vi "Tactic.vi"(11 "IA State Input":T1) -> (3 "IA State Output":T1)   [LabVIEW 2016]
uses:
  Core/AI Input.ctl
  Core/AI Robot.ctl
  Core/AI Ball.ctl
  Core/Field Size.ctl
  Core/AI Judge.ctl
  Command Enum.ctl
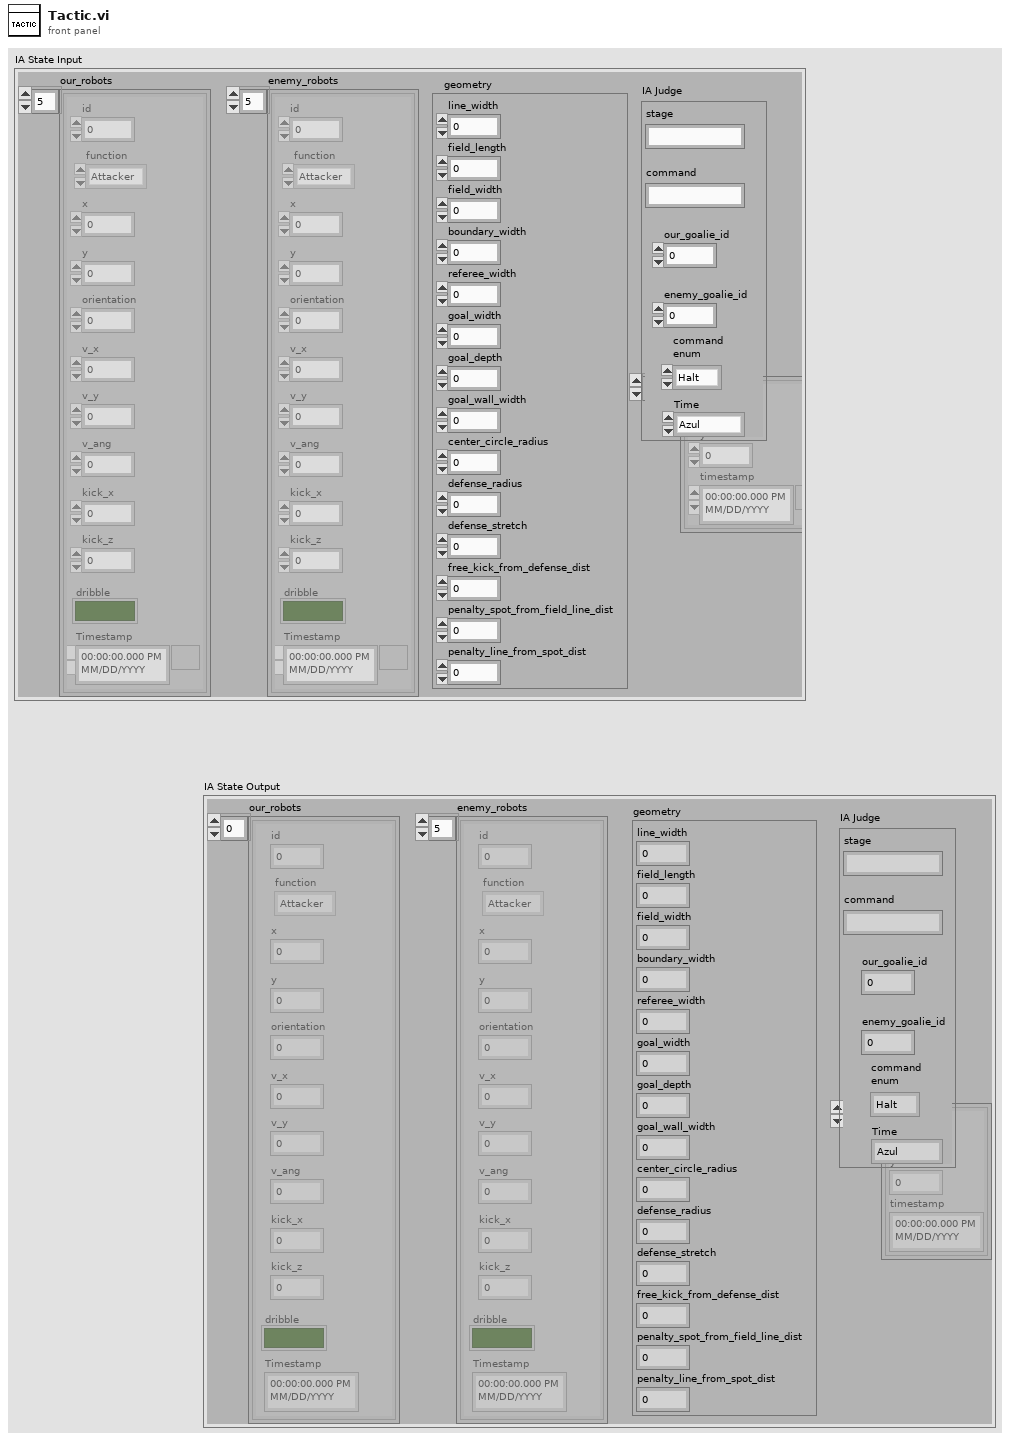
[diagram p1: front panel]
types:
  T1 = typedef "AI Input.ctl" = cluster{"our_robots":T2[], "enemy_robots":T2[], "balls":T3[], "geometry":T4, "IA Judge":T5}
  T2 = typedef "AI Robot.ctl" = cluster{"id":u32, "function":enum16{"Attacker", "Goalie", "Defender"}, "x":dbl, "y":dbl, "orientation":dbl, "v_x":dbl, "v_y":dbl, "v_ang":dbl, "kick_x":dbl, "kick_z":dbl, "dribble":bool, "Timestamp":timestamp}
  T3 = typedef "AI Ball.ctl" = cluster{"x":dbl, "y":dbl, "timestamp":timestamp}
  T4 = typedef "Field Size.ctl" = cluster{"line_width":u32, "field_length":u32, "field_width":u32, "boundary_width":u32, "referee_width":u32, "goal_width":u32, "goal_depth":u32, "goal_wall_width":u32, "center_circle_radius":u32, "defense_radius":u32, "defense_stretch":u32, "free_kick_from_defense_dist":u32, "penalty_spot_from_field_line_dist":u32, "penalty_line_from_spot_dist":u32}
  T5 = typedef "AI Judge.ctl" = cluster{"stage":string, "command":string, "our_goalie_id":dbl, "enemy_goalie_id":dbl, "command\nenum":T6, "Time":enum16{"Azul", "Amarelo"}}
  T6 = typedef "Command Enum.ctl" = enum16{"Halt", "Stop", "Force Start", "PKA Normal Start", "Prepare Kickoff Ally", "PKE Normal Start", "Prepare Kickoff Enemy", "Prepare Penalty Ally", "Prepare Penalty Enemy", "Direct Free Enemy", "Direct Free Ally", "Indirect Free Enemy", "Indirect Free Ally", "Timeout Enemy", "Timeout Ally", "Goal Enemy", "Goal Ally", "Ball Placement Enemy", "Ball Placement Ally", "None"}
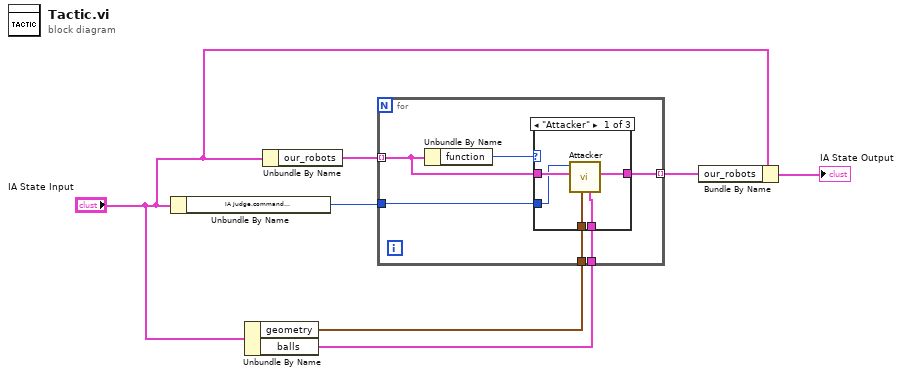
[diagram p0: block diagram]
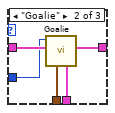
[diagram p2: hidden frame]
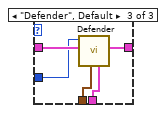
[diagram p3: hidden frame]
diagram:
  n1 = Unbundle By Name("IA State Input") -> ("IA Judge.command\nenum"=w6:T6)
  n2 = Unbundle By Name("IA State Input") -> ("geometry"=w2:T4, "balls"=w1:T3[])
  n3 = Unbundle By Name("IA State Input") -> ("our_robots"=w7:T2[])
  n4 = for {
    tunnel: w7 -> [w12] mode=indexing
    tunnel: [w11] -> w5 mode=indexing
    tunnel: w6 -> [w10]
    tunnel: w2 -> [w9]
    tunnel: w1 -> [w8]
    n5 = Unbundle By Name(w12) -> ("function"=w13:enum16{"Attacker", "Goalie", "Defender"})
    n6 = case shown="\"Attacker\"" w13 {
      tunnel: w12 -> [w18 w23 w28]
      tunnel: [w17 w22 w26] -> w11
      tunnel: w10 -> [w16 w21 w27]
      tunnel: w9 -> [w15 w19 w24]
      tunnel: w8 -> [w14 w20 w25]
      frame "Attacker" {
        n7 = call "Attacker.vi"("balls"=w14, "Field Size 2"=w15, "Robot"=w18, "command\nenum"=w16) -> ("output cluster"=w17:T2)  [unwired: 7 in]
      }
      frame "Goalie" {
        n8 = call "Goalie.vi"("balls"=w20, "Field Size 2"=w19, "Robot"=w23, "command\nenum"=w21) -> ("output cluster"=w22:T2)  [unwired: 7 in]
      }
      frame "Defender", Default {
        n9 = call "Defender.vi"("balls"=w25, "Field Size 2"=w24, "Robot"=w28, "command\nenum"=w27) -> ("output cluster"=w26:T2)  [unwired: 7 in]
      }
    }
  }
  n10 = Bundle By Name(cluster="IA State Input", "our_robots"=w5) -> (→"IA State Output":T1)
